vi "Found shot match utility.vi"(7 "Log file folder":path=path "C:/Data", 8 "error in (no error)":errorcluster, 9 "Shot data":T1, 10 "Idot match record":T2, 11 "Root Data Folder":path=path "C:/Data") -> (0 "error out":errorcluster, 2 "Formated shot data":string, 3 "File output":path)   [LabVIEW 2015]
uses:
  Mag Lab Measure/Mag Lab Measure Controller/Cap Bank Server/Idot match record.ctl
  Shot data.ctl
  File/Controls/File formats.ctl
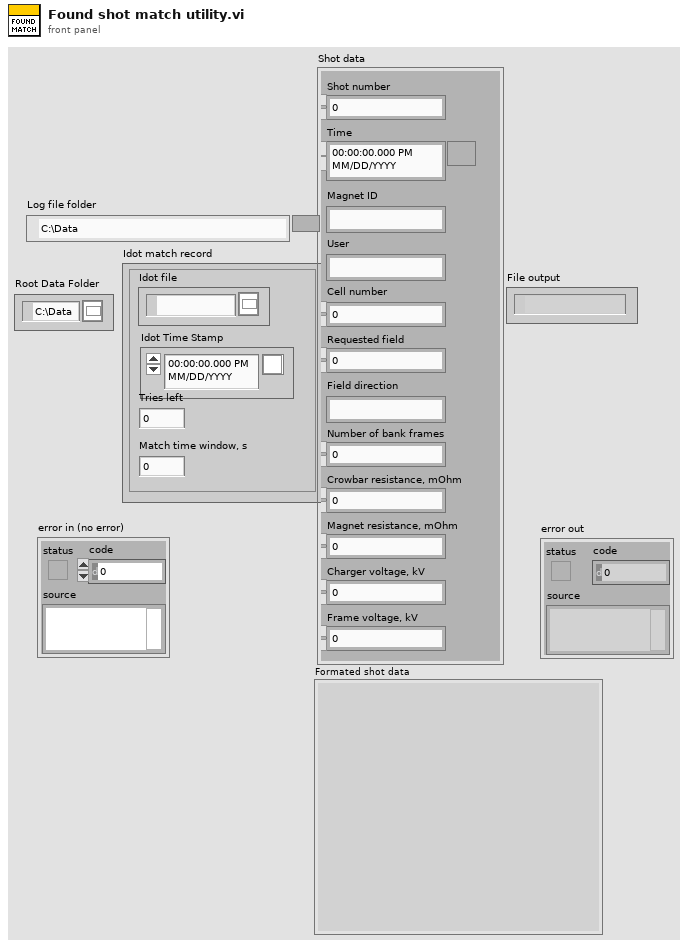
[diagram p1: front panel]
types:
  T1 = typedef "Shot data.ctl" = cluster{"Shot number":i32, "Time":timestamp, "Magnet ID":string, "User":string, "Cell number":i32, "Requested field":dbl, "Field direction":string, "Number of bank frames":i32, "Crowbar resistance, mOhm":dbl, "Magnet resistance, mOhm":dbl, "Charger voltage, kV":dbl, "Frame voltage, kV":dbl}
  T2 = typedef "Idot match record.ctl" = cluster{"Idot file":path, "Idot Time Stamp":timestamp, "Tries left":i32, "Match time window, s":dbl}
  T3 = typedef "File formats.ctl" = enum16{"TDMS", "ASCII", "BINARY"}
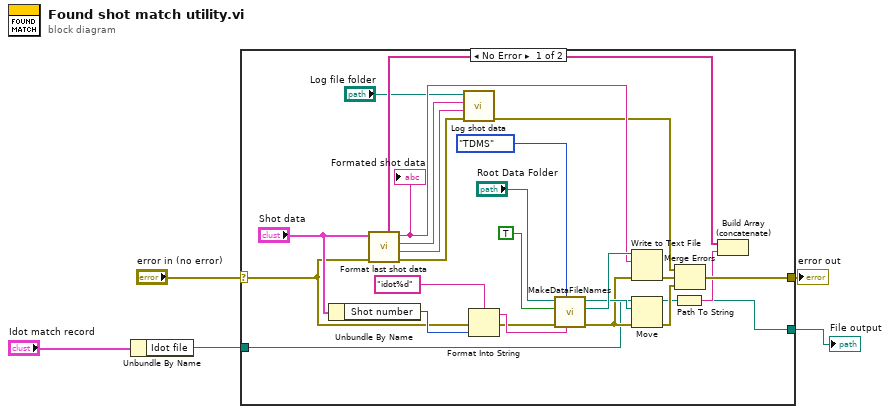
[diagram p0: block diagram]
diagram:
  n1 = Unbundle By Name("Idot match record") -> ("Idot file"=w2:path)
  n2 = case shown="No Error" "error in (no error)" {
    selector: "error in (no error)" -> [w10 w32]
    tunnel: [w16 w32] -> w4
    tunnel: w2 -> [w7 w31]
    tunnel: [w6 w31] -> w1
    frame No Error {
      n3 = Unbundle By Name("Shot data") -> ("Shot number"=w21:i32)
      n4 = call "Format last shot data.vi"("error in (no error)"=w10, "Shot data"="Shot data") -> ("error out"=w12:errorcluster, "Spreadsheet header string"=w23:string, "Spreadsheet shot string"=w24:string, "Formated shot data"=w25:string, "Listbox entry"=w15:string[])  [unwired: 5 in]
      "Formated shot data" <- w25
      n5 = call "Log shot data.vi"("error in (no error)"=w12, "Spreadsheet header string"=w23, "Spreadsheet shot string"=w24, "Log file folder"="Log file folder") -> ("error out"=w11:errorcluster)  [unwired: 6 in, 1 out]
      n6 = Format Into String(format string="idot%d", error in=w10, w21) -> (resulting string=w28:string, error out=w22:errorcluster)  [unwired: 1 in]
      n7 = call "MakeDataFileNames.vi"("File Prefix"=w28, "File format"=File_formats."TDMS", "Error In"=w22, "Generate Index"=TRUE, "Root Data Folder"="Root Data Folder") -> ("Error Out"=w13:errorcluster, "Settings File Path"=w26:path, "Data File  Path"=w20:path)  [unwired: 3 in, 1 out]
      n8 = Write to Text File(file (use dialog)=w26, text=w25, error in=w13) -> (error out=w18:errorcluster)  [unwired: 1 in, 2 out]
      n9 = Move(source path=w7, error in=w13, 10:w20) -> (error out=w17:errorcluster, 3:w6:path)  [unwired: 2 in, 1 out]
      n10 = Path To String(path=w6) -> (string=w14:string)
      n11 = Merge Errors(w11, w18, w17) -> (w16:errorcluster)
      n12 = Build Array (concatenate)(w15, w14) -> ()  [unwired: 1 out]
    }
    frame Error {
    }
  }
  "error out" <- w4
  "File output" <- w1
